vi "Init Headers.vi"(5 "httpHeaders in":refnum<class "httpHeaders.lvclass">, 10 "headers":cluster{"header":string, "value":string}[](array[cluster]), 11 "http-header (unparsed)":string) -> (3 "httpHeaders out":refnum<class "httpHeaders.lvclass">)   [LabVIEW 2020, in "httpClient.lvlib" / "httpHeaders.lvclass"]
uses:
  httpHeaders.lvclass
  httpHeaders.lvclass/httpHeaders.ctl
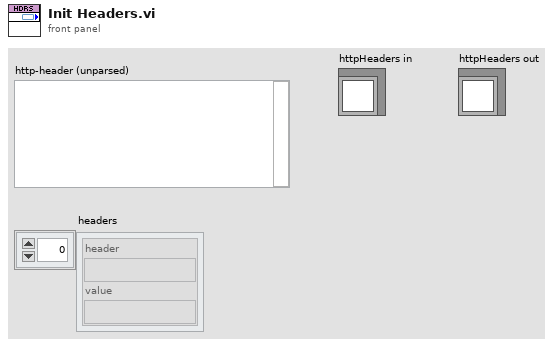
[diagram p1: front panel]
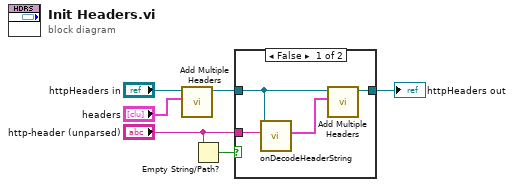
[diagram p0: block diagram]
diagram:
  n1 = call "Add Multiple Headers.vi"("headers"="headers", "httpHeaders in"="httpHeaders in") -> ("httpHeaders out"=w1:refnum<class "httpHeaders.lvclass">)  [unwired: 8 in, 1 out]
  n2 = Empty String/Path?(string/path="http-header (unparsed)") -> (empty?=w5:bool)
  n3 = case shown="False" w5 {
    tunnel: "http-header (unparsed)" -> [w7 _]
    tunnel: w1 -> [w8 w11]
    tunnel: [w10 w11] -> w4
    frame False {
      n4 = call-dynamic "onDecodeHeaderString.vi"("http-header (unparsed)"=w7, "httpHeaders"=w8) -> ("headers"=w9:cluster{"header":string, "value":string}[])  [unwired: 8 in, 1 out]
      n5 = call "Add Multiple Headers.vi"("headers"=w9, "httpHeaders in"=w8) -> ("httpHeaders out"=w10:refnum<class "httpHeaders.lvclass">)  [unwired: 8 in, 1 out]
    }
    frame True {
    }
  }
  "httpHeaders out" <- w4
